vi "waitForAllIRQs.vi"(8 "error in (no error)":errorcluster, 10 "Timeout":i32, 11 "ILCCommunications in":refnum<class "ILCCommunications.lvclass">) -> (0 "error out":errorcluster, 3 "ILCCommunications out":refnum<class "ILCCommunications.lvclass">)   [LabVIEW 2016, in "ILCCommunications.lvclass"]
uses:
  ILCCommunications.lvclass
  ILCCommunications.lvclass/ILCCommunications.ctl
  Common_RT_FPGA/IIRQ/IIRQ.lvclass
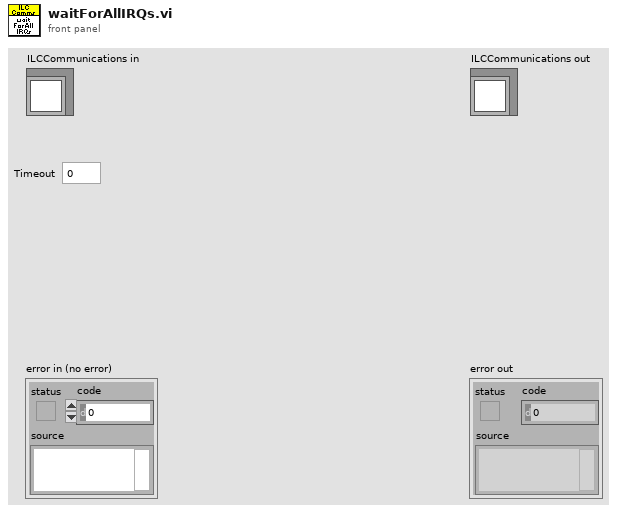
[diagram p1: front panel]
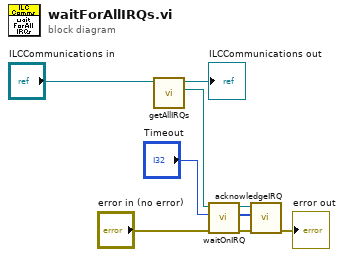
[diagram p0: block diagram]
diagram:
  n1 = call "getAllIRQs.vi"("ILCCommunications in"="ILCCommunications in") -> ("AllIRQs"=w8:refnum<class "IIRQ.lvclass">, "ILCCommunications out"=→"ILCCommunications out":refnum<class "ILCCommunications.lvclass">)  [unwired: 9 in]
  n2 = call-dynamic "waitOnIRQ.vi"("error in (no error)"="error in (no error)", "Timeout"="Timeout", "IIRQ in"=w8) -> ("error out"=w4:errorcluster, "IRQs"=w6:i32[], "IIRQ out"=w5:refnum<class "IIRQ.lvclass">)  [unwired: 5 in, 1 out]
  n3 = call-dynamic "acknowledgeIRQ.vi"("error in (no error)"=w4, "IRQs"=w6, "IIRQ in"=w5) -> ("error out"=→"error out":errorcluster)  [unwired: 7 in, 1 out]
